vi "Exemple de mesure.vi"() -> ()   [LabVIEW 2013]
panel:
  out "error out":errorcluster
  out "XY Graph":cluster{dbl[], dbl[]}(graph)
  out "P1/P2":dbl format="%#_13g"
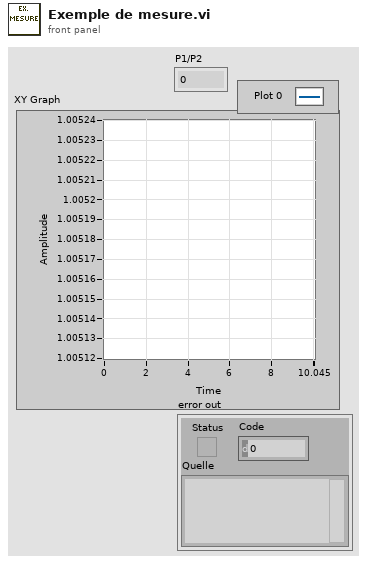
[diagram p1: front panel]
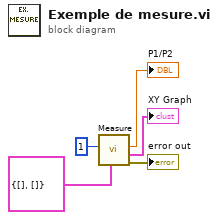
[diagram p0: block diagram]
diagram:
  n1 = call "Measure.vi"("Graph in"=cluster{dbl[], dbl[]} {[], []}, "Reference Cell"=1) -> ("error out"=→"error out":errorcluster, "Values"=→"XY Graph":cluster{dbl[], dbl[]}, "P1/P2"=→"P1/P2":dbl)  [unwired: 7 in]
